vi "PhaseShifter demo init.vi"() -> (0 "Error Out":errorcluster, 1 "De-embedding files":path[](array[path]), 2 "Toggle 6.lvclass":refnum<class "Toggle 6.lvclass">, 3 "Vector Network Analyzer.lvclass":refnum<class "Vector Network Analyzer.lvclass">, 4 "Cancelled":bool, 6 "VNA ports 2":bool[](array[boolean])=[FALSE, FALSE, TRUE, TRUE])   [LabVIEW 2020]
uses:
  Instruments/Vector Network Analyzer/Vector Network Analyzer.lvclass
  C:/Sandbox/RF Bench/Source Code/WiSpry Test Framework/Instruments/Instrument.lvclass
  Devices/Toggle 6/Toggle 6.lvclass
  Instruments/Instrument.lvclass/Instrument.ctl
  Instruments/Instrument.lvclass
panel:
  in  "Channel":i32=2
  in  "VNA ports":bool[](array[boolean])=[FALSE, FALSE, TRUE, TRUE]
  in  "WS104x VISA address":refnum<visa-resource-name>
  in  "Cancel Button":bool
  in  "OK Button":bool
  in  "De-embedding files":path[](array[path])=[path "", path ""]
  in  "VNA model":u16(ring)=3 items=["Ag87xx", "CMT S2 S4", "FieldFox", "Keysight PNA", "PNA", "ZNB"]
  out "Array":string[](array[string])
  in  "VNA VISA address":refnum<visa-resource-name>
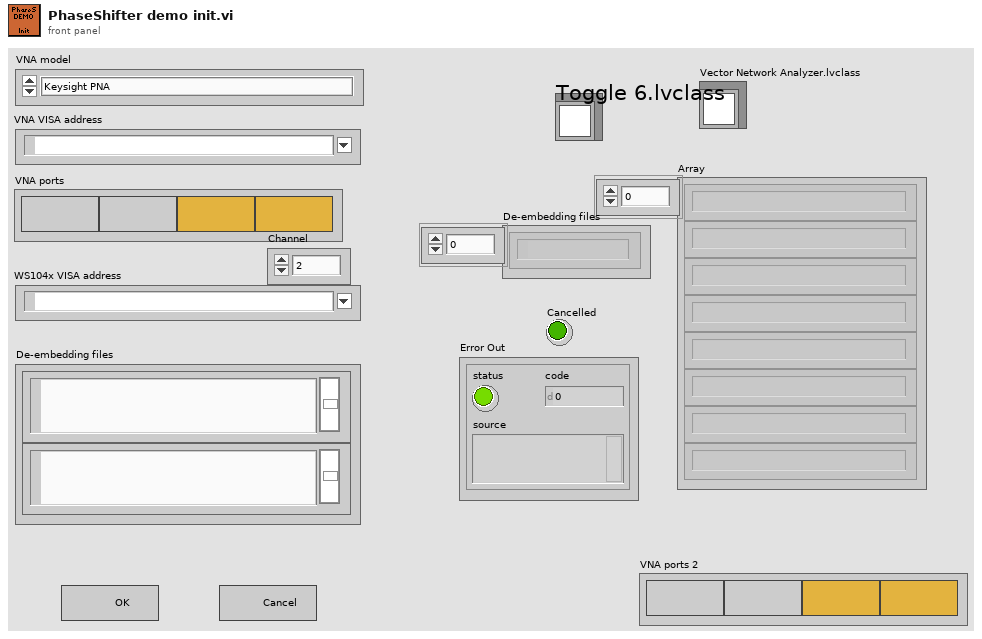
[diagram p1: front panel]
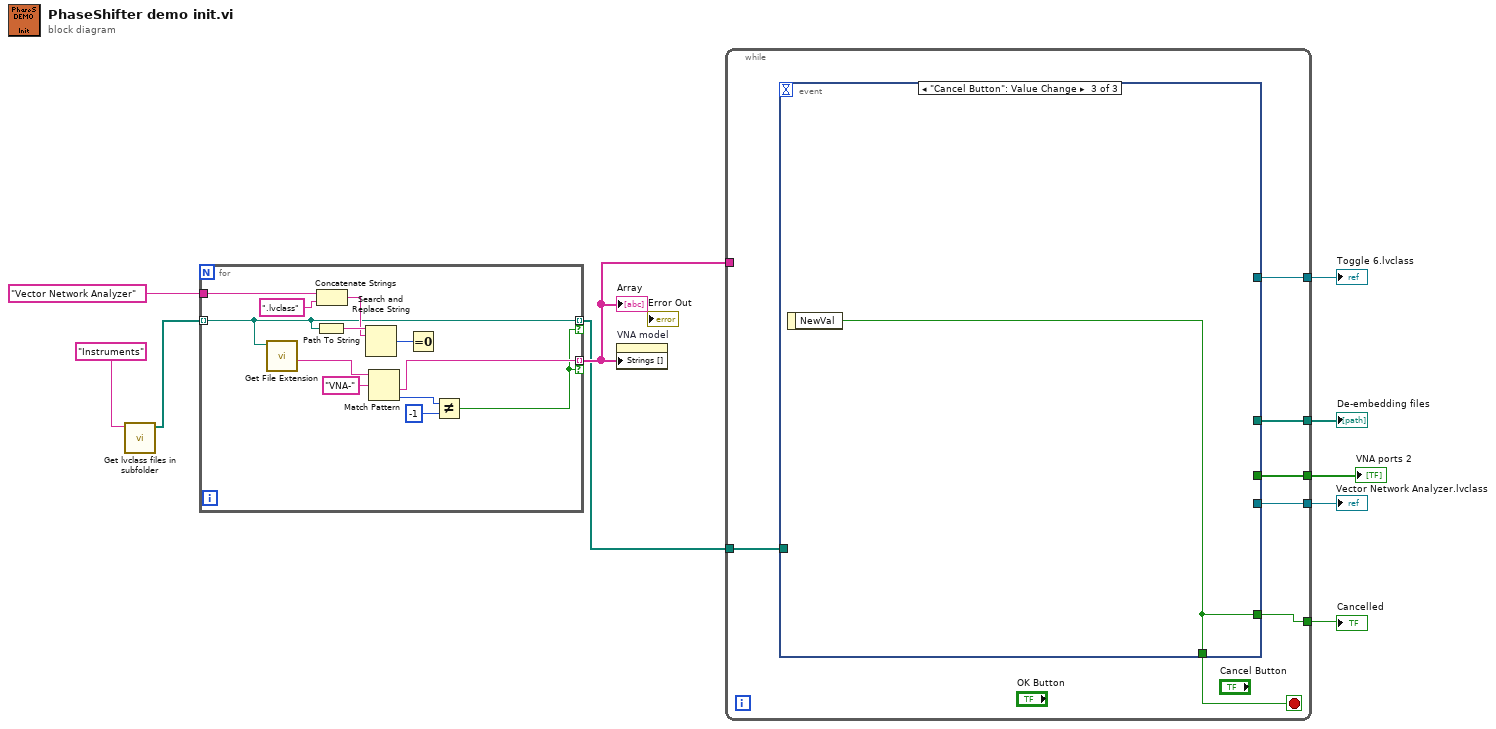
[diagram p0: block diagram]
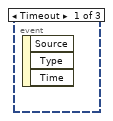
[diagram p2: hidden frame]
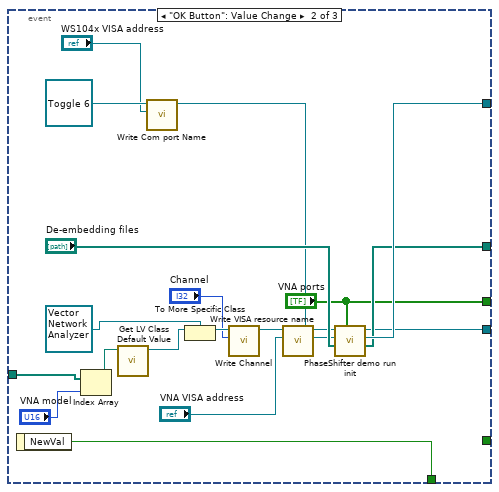
[diagram p3: hidden frame]
diagram:
  n1 = call "Get lvclass files in subfolder.vi"("Sub Folder"="Instruments") -> ("Found lvclass files"=w9:path[])  [unwired: 9 in, 1 out]
  n2 = for {
    tunnel: w9 -> [w17] mode=indexing
    tunnel: "Vector Network Analyzer" ("Sub Folder") -> [w20]
    tunnel: [w17] -> w2 mode=indexing if=w11
    tunnel: [w14] -> w7 mode=indexing if=w11
    n3 = call <vilib>:"Get File Extension.vi"("file"=w17) -> ("filename without extension"=w16:string)  [unwired: 6 in, 4 out]
    n4 = Path To String(path=w17) -> (string=w22:string)
    n5 = Concatenate Strings(w20, ".lvclass" ("string")) -> (w21:string)
    n6 = Search and Replace String(input string=w22, search string=w21) -> (number of replacements=w18:i32)  [unwired: 6 in, 3 out]
    n7 = Match Pattern(string=w16, regular expression="VNA-") -> (after substring=w14:string, offset past match=w12:i32)  [unwired: 1 in, 2 out]
    n8 = Equal To 0?(x=w18) -> ()  [unwired: 1 out]
    n9 = Not Equal?(x=w12, y=-1) -> (x != y?=w11:bool)
  }
  "Array" <- w7
  n10 = property on="VNA model" class="Ring (strict)"("Strings []"=w7) -> ()  [unwired: 2 in, 2 out]
  n11 = while {
    tunnel: w7 -> [_]
    tunnel: [w28] -> w6
    tunnel: [w27] -> w5
    tunnel: [w23] -> w4
    tunnel: [w26] -> w3
    tunnel: w2 -> [w25]
    tunnel: [w24] -> w1
    stop <- w29 stop-if-true
    n12 = event shown="[2] \"Cancel Button\": Value Change" {
      selector: _ -> [_ _ _]
      dyn-events: _ -> [_ _ _]
      timeout: _ -> [_ _ _]
      tunnel: [_ w48 w49] -> w29
      tunnel: [_ w41 _] -> w28
      tunnel: [_ w39 _] -> w27
      tunnel: [_ w42 _] -> w26
      tunnel: w25 -> [_ w38 _]
      tunnel: [_ "VNA ports" _] -> w24
      tunnel: [_ _ w49] -> w23
      event Timeout {
        n13 = event-data() -> ()  [unwired: 1 in, 3 out]
      }
      event "OK Button": Value Change {
        n14 = event-data() -> ("NewVal"=w48:bool)  [unwired: 1 in]
        n15 = Index Array(array=w38, index="VNA model") -> (element=w36:path)
        n16 = call <vilib>:"Get LV Class Default Value.vi"("class path"=w36) -> ("object"=w35:refnum<class>)  [unwired: 9 in, 1 out]
        n17 = call-dynamic "Write Com port Name.vi"("Com port Name"="WS104x VISA address", "Device in"=refnum<class "Toggle 6.lvclass"> refnum ("Toggle 6.lvclass")) -> ("Device out"=w43:refnum<class "Toggle 6.lvclass">)  [unwired: 9 in]
        n18 = To More Specific Class(target class=refnum<class "Vector Network Analyzer.lvclass"> refnum ("Vector Network Analyzer.lvclass"), reference=w35) -> (specific class reference=w32:refnum<class "Vector Network Analyzer.lvclass">)  [unwired: 1 in, 1 out]
        n19 = call-dynamic "Write Channel.vi"("Channel"="Channel", "Vector Network Analyzer in"=w32) -> ("Vector Network Analyzer out"=w31:refnum<class "Vector Network Analyzer.lvclass">)  [unwired: 9 in]
        n20 = call "Write VISA resource name.vi"("VISA resource name"="VNA VISA address", "Instrument in"=w31) -> ("Instrument out"=w40:refnum<class "Vector Network Analyzer.lvclass">)  [unwired: 9 in]
        n21 = call "PhaseShifter demo run init.vi"("VNA ports"="VNA ports", "De-embedding files in"="De-embedding files", "Toggle 6.lvclass in"=w43, "Vector Network Analyzer.lvclass in"=w40) -> ("De-embedding files"=w41:path[], "Toggle 6.lvclass"=w42:refnum<class "Toggle 6.lvclass">, "Vector Network Analyzer.lvclass"=w39:refnum<class "Vector Network Analyzer.lvclass">)  [unwired: 5 in]
      }
      event "Cancel Button": Value Change {
        n22 = event-data() -> ("NewVal"=w49:bool)  [unwired: 1 in]
      }
    }
  }
  "De-embedding files" <- w6
  "Vector Network Analyzer.lvclass" <- w5
  "Cancelled" <- w4
  "Toggle 6.lvclass" <- w3
  "VNA ports 2" <- w1
